vi "Open Block Diagram.vi"(8 "error in (no error)":errorcluster, 11 "VI Refnum":refnum<vi>) -> (0 "error out (no error)":errorcluster, 3 "reference out":refnum<vi>)   [LabVIEW 2014]
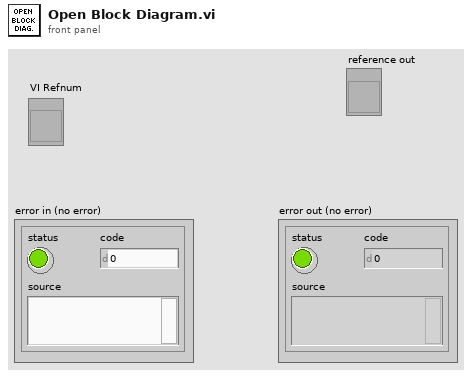
[diagram p1: front panel]
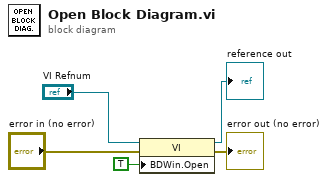
[diagram p0: block diagram]
diagram:
  n1 = property class="VI"(reference="VI Refnum", error in="error in (no error)", "BDWin.Open"=TRUE ("Block Diagram Window:Open")) -> (reference out=→"reference out":refnum<vi>, error out=→"error out (no error)":errorcluster)
